vi "evaluateGenerateXML.vi"(8 "error in":errorcluster, 9 "Input Data":variant, 11 "reference in":refnum<class "EasyXML_XML_Subset_Evaluations.lvclass">) -> (0 "error out":errorcluster, 1 "XML String":string, 3 "reference out":refnum<class "EasyXML_XML_Subset_Evaluations.lvclass">)   [LabVIEW 2011, in "EasyXML_XML_Subset_Evaluations.lvclass"]
uses:
  EasyXML_XML_Subset_Evaluations.lvclass
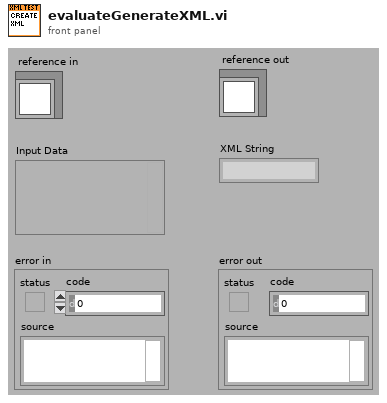
[diagram p1: front panel]
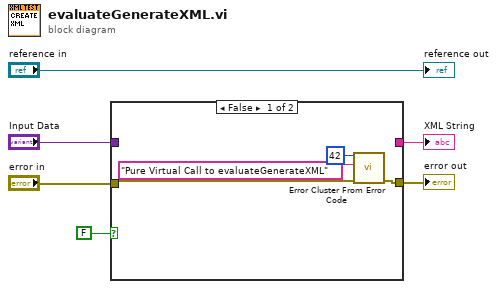
[diagram p0: block diagram]
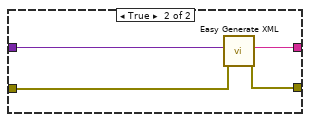
[diagram p2: hidden frame]
diagram:
  n1 = case shown="False" FALSE {
    tunnel: [_ w14] -> w5
    tunnel: [w7 w13] -> w4
    tunnel: "error in" -> [w8 w12]
    tunnel: "Input Data" -> [_ w11]
    frame False {
      n2 = call <vilib>:"Error Cluster From Error Code.vi"("error in (no error)"=w8, "error message (\"\")"="Pure Virtual Call to evaluateGenerateXML" ("error message (\"\")"), "error code (0)"=42) -> ("error out"=w7:errorcluster)  [unwired: 6 in]
    }
    frame True {
      n3 = call "Easy Generate XML.vi"("error in (no error)"=w12, "LabVIEW Data"=w11) -> ("error out"=w13:errorcluster, "XML String"=w14:string)  [unwired: 8 in]
    }
  }
  "XML String" <- w5
  "error out" <- w4
  "reference out" <- "reference in"
